vi "Disconnect.vi"(8 "error in":errorcluster, 11 "2525 in":refnum<class "2525.lvclass">) -> (0 "error out":errorcluster, 3 "2525 out":refnum<class "2525.lvclass">)   [LabVIEW 2019, in "2525.lvlib" / "2525.lvclass"]
doc: "Override VI, close communication with the instrument and cleanly destroy the resource reference."
uses:
  Library/2525.lvclass
  Library/2525.lvclass/2525.ctl
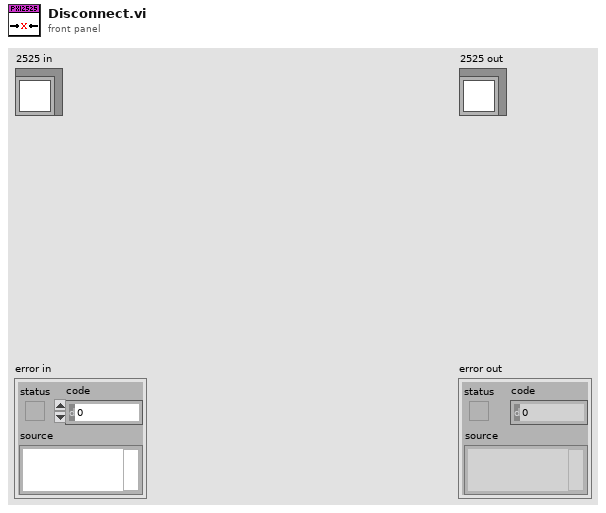
[diagram p1: front panel]
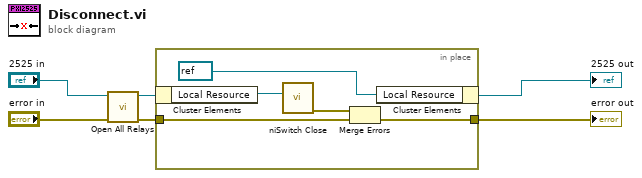
[diagram p0: block diagram]
diagram:
  n1 = call-dynamic "Open All Relays.vi"("error in"="error in", "2525 in"="2525 in") -> ("error out"=w2:errorcluster, "2525 out"=w4:refnum<class "2525.lvclass">)  [unwired: 8 in]
  n2 = in-place {
    in-place-border: w2 -> [w8]
    in-place-border: [w7] -> w1
    n3 = in-place-cluster #1(w4) -> ("Local Resource"=w11:refnum<k15>)
    n4 = call <instrlib>:"niSwitch Close.vi"("instrument handle"=w11) -> ("error out"=w9:errorcluster)  [unwired: 10 in]
    n5 = Merge Errors(w9, w8) -> (w7:errorcluster)
    n6 = in-place-cluster #1("Local Resource"=refnum<k15> refnum) -> (→"2525 out":refnum<class "2525.lvclass">)
  }
  "error out" <- w1
